vi "Autodetect SLSC Module Name.vi"(8 "error in (no error)":errorcluster, 11 "Item Ref in":T1 format="%.0x") -> (0 "error out":errorcluster, 2 "SLSC Module Name":refnum<k21>, 3 "Item Ref out":T1 format="%.0x")   [LabVIEW 2017, in "SLSC Switch Scripting.lvlib"]
uses:
  SLSC Switch Scripting.lvlib
  <vilib>/NI Veristand/Custom Device API/Custom Device Item Ref.ctl
  <vilib>/NI Veristand/Custom Device API/Get Item Property (I32).vi
  <vilib>/nisyscfg/Close (System).vi
  <vilib>/SLSC/Initialize Session with Devices.vi
  <vilib>/SLSC/Close Session.vi
  <vilib>/nisyscfg/nisyscfg.lvlib
  <resource>/objmgr/nisysapi.rc
  <vilib>/SLSC/SLSC.lvlib
  <resource>/objmgr/slsc.rc
  <vilib>/NI Veristand/Custom Device API/Custom Device API.lvlib
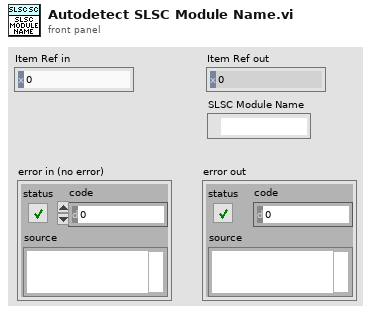
[diagram p1: front panel]
types:
  T1 = typedef "Custom Device API.lvlib/Custom Device Item Ref.ctl" = u64
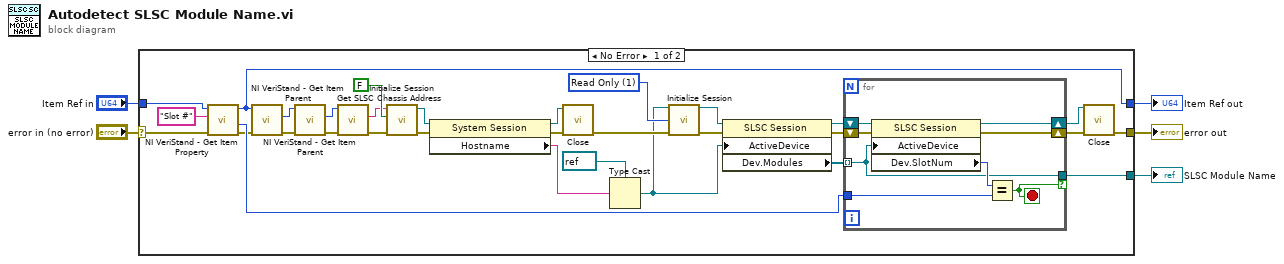
[diagram p0: block diagram]
diagram:
  n1 = case shown="No Error" "error in (no error)" {
    selector: "error in (no error)" -> [w22 w46]
    tunnel: [w20 _] -> w4
    tunnel: "Item Ref in" -> [w19 w45]
    tunnel: [w16 w46] -> w2
    tunnel: [w8 w45] -> w1
    frame No Error {
      w31 = 1 items=["None"=0, "Read Only"=1, "Read/Write"=3] ("reservation access (Read/Write)")
      n2 = call-poly <vilib>:"NI VeriStand - Get Item Property.vi"("error in (no error)"=w22, "Property Name"="Slot #", "Item Ref in"=w19) -> ("error out"=w9:errorcluster, "Value"=w21:i32, "Item Ref out"=w8:T1)  [unwired: 5 in, 1 out]
      n3 = call <vilib>:"NI VeriStand - Get Item Parent.vi"("error in (no error)"=w9, "Item Ref in"=w8) -> ("error out"=w10:errorcluster, "Parent Ref"=w7:T1)  [unwired: 6 in, 2 out]
      n4 = call <vilib>:"NI VeriStand - Get Item Parent.vi"("error in (no error)"=w10, "Item Ref in"=w7) -> ("error out"=w11:errorcluster, "Parent Ref"=w6:T1)  [unwired: 6 in, 2 out]
      n5 = call "Get SLSC Chassis Address.vi"("error in (no error)"=w11, "SLSC Chassis Ref in"=w6) -> ("error out"=w15:errorcluster, "IP Address"=w14:string)  [unwired: 6 in, 2 out]
      n6 = call <vilib>:"Initialize Session.vi"("error in (no error)"=w15, "Force Property Refresh (T)"=FALSE, "Target (localhost)"=w14) -> ("error out"=w35:errorcluster, "Session out"=w36:refnum<k21>)  [unwired: 7 in]
      n7 = property class="System Session"(reference=w36, error in=w35) -> (reference out=w32:refnum<k21>, error out=w34:errorcluster, "Hostname"=w13:string)
      n8 = call-poly <vilib>:"Close.vi"("error in (no error)"=w34, "Session in"=w32) -> ("error out"=w30:errorcluster)  [unwired: 9 in]
      n9 = Type Cast(type=refnum<k21> refnum ("devices"), x=w13) -> (*(type *) &x=w26:refnum<k21>)
      n10 = call-poly <vilib>:"Initialize Session.vi"("devices"=w26, "reservation access (Read/Write)"=w31, "error in (no error)"=w30) -> ("session out"=w29:refnum<k21>, "error out"=w28:errorcluster)  [unwired: 11 in]
      n11 = property class="SLSC Session"(reference=w29, error in=w28, "ActiveDevice"=w26) -> (reference out=w25:refnum<k21>, error out=w24:errorcluster, "Dev.Modules"=w12:refnum<k21>[])
      n12 = for {
        tunnel: w12 -> [w38] mode=indexing
        shift-right: [w42] -> w17
        shift-left: w24 -> [w43]
        shift-right: [w41] -> w18
        shift-left: w25 -> [w44]
        tunnel: w21 -> [w39]
        tunnel: [w38] -> w20 if=w37
        stop <- w37 stop-if-true
        n13 = property class="SLSC Session"(reference=w44, error in=w43, "ActiveDevice"=w38) -> (reference out=w41:refnum<k21>, error out=w42:errorcluster, "Dev.SlotNum"=w40:u32)
        n14 = Equal?(x=w40, y=w39) -> (x = y?=w37:bool)
      }
      n15 = call-poly <vilib>:"Close.vi"("session in"=w18, "error in (no error)"=w17) -> ("error out"=w16:errorcluster)  [unwired: 13 in]
    }
    frame Error {
    }
  }
  "SLSC Module Name" <- w4
  "Item Ref out" <- w1
  "error out" <- w2
